vi "getViLogEvent.vi"(8 "error in (no error)":errorcluster, 10 "name":string, 11 "LibReader in":refnum<class "LibReader.lvclass">) -> (0 "error out":errorcluster, 1 "clusterNameInput":string, 2 "pathViLogEvent":path, 3 "LibReader out":refnum<class "LibReader.lvclass">)   [LabVIEW 2018, in "LibReader.lvclass"]
doc: "Get the path of log event vi."
uses:
  LibReader.lvclass
  LibReader.lvclass/LibReader.ctl
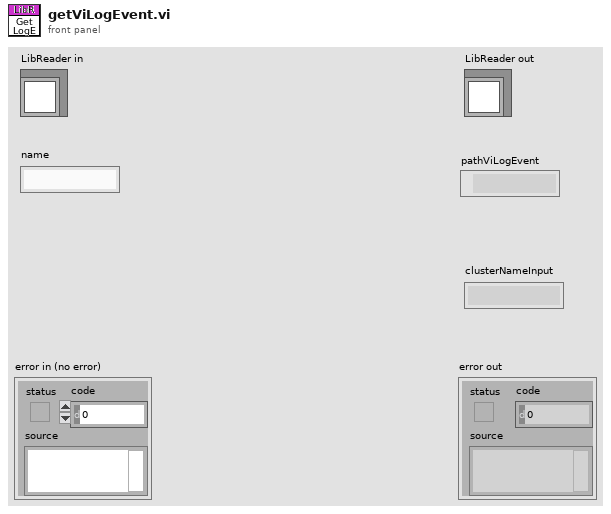
[diagram p1: front panel]
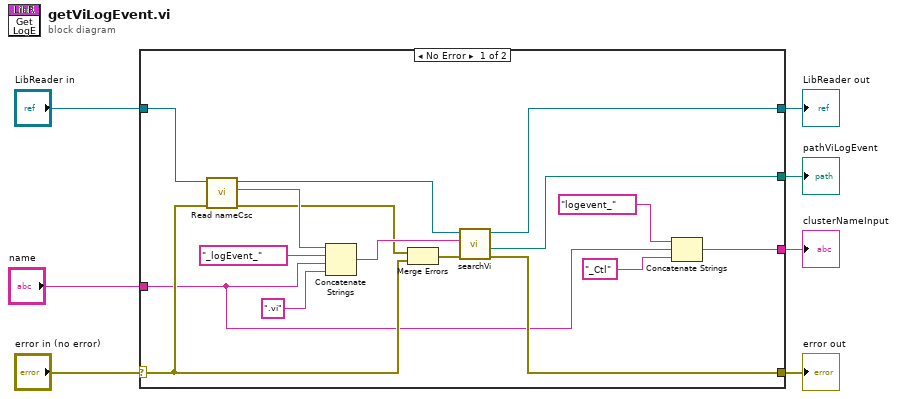
[diagram p0: block diagram]
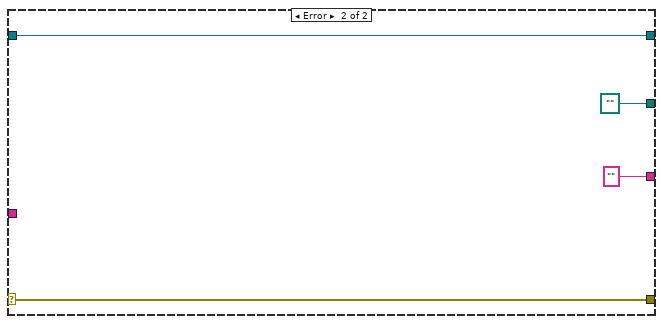
[diagram p2: hidden frame]
diagram:
  n1 = case shown="No Error" "error in (no error)" {
    selector: "error in (no error)" -> [w15 w27]
    tunnel: [w14 w27] -> w6
    tunnel: [w12 w26] -> w4
    tunnel: "LibReader in" -> [w18 w26]
    tunnel: [w23 path "" ("pathVi")] -> w3
    tunnel: "name" -> [w10 _]
    tunnel: [w8 ""] -> w1
    frame No Error {
      n2 = call "Read nameCsc.vi"("error in (no error)"=w15, "LibReader in"=w18) -> ("error out"=w17:errorcluster, "nameCsc"=w19:string, "LibReader out"=w13:refnum<class "LibReader.lvclass">)  [unwired: 7 in]
      n3 = Concatenate Strings(w19, "_logEvent_" ("regExpr"), w10, ".vi" ("regExpr")) -> (w20:string)
      n4 = Merge Errors(w17, w15) -> (w16:errorcluster)
      n5 = call "searchVi.vi"("error in (no error)"=w16, "regExpr"=w20, "LibReader in"=w13) -> ("error out"=w14:errorcluster, "pathVi"=w23:path, "LibReader out"=w12:refnum<class "LibReader.lvclass">)  [unwired: 5 in, 1 out]
      n6 = Concatenate Strings("logevent_", w10, "_Ctl") -> (w8:string)
    }
    frame Error {
    }
  }
  "error out" <- w6
  "LibReader out" <- w4
  "pathViLogEvent" <- w3
  "clusterNameInput" <- w1
